vi "Telnet Parse AIC Command.vi"(11 "AIC sequence":string) -> (0 "error":bool, 1 "command":string, 2 "after sequence":string, 3 "AIC result":string, 4 "option negotiation":bool, 5 "sub option negotiation":bool, 6 "option info":T1)   [LabVIEW 2015, in "NI_InternetTK_Core_VIs.lvlib"]
uses:
  NI_InternetTK_Core_VIs.lvlib
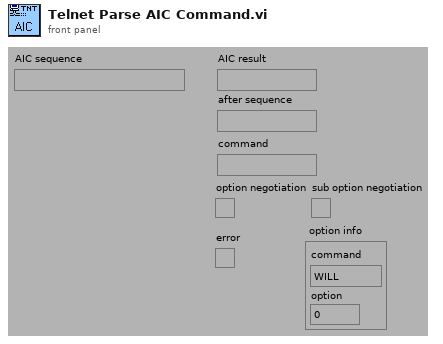
[diagram p1: front panel]
types:
  T1 = cluster{"command":enum16{"WILL", "WON'T", "DO", "DON'T"}, "option":u8}
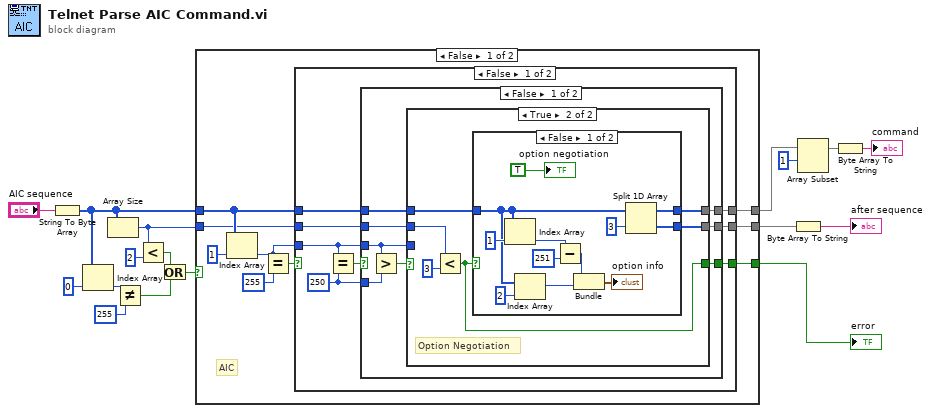
[diagram p0: block diagram]
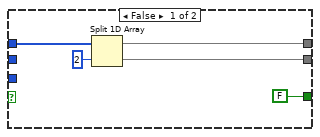
[diagram p2: hidden frame]
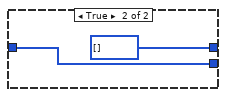
[diagram p3: hidden frame]
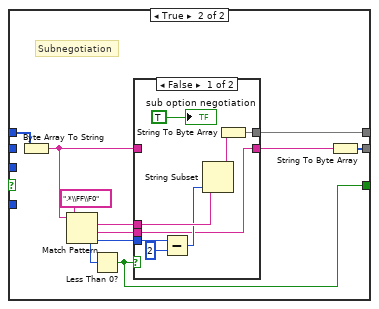
[diagram p4: hidden frame]
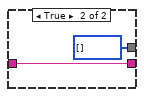
[diagram p5: hidden frame]
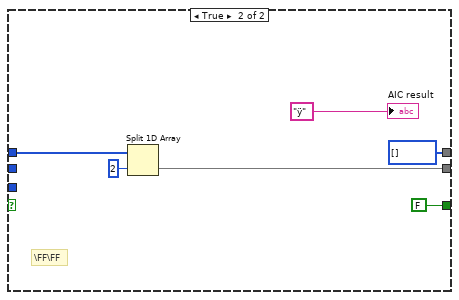
[diagram p6: hidden frame]
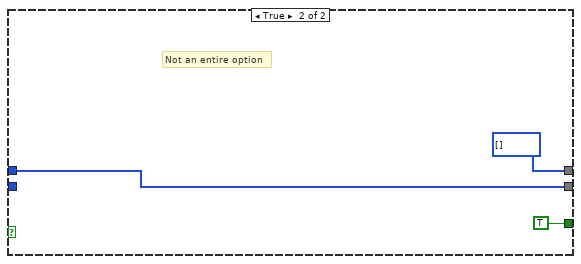
[diagram p7: hidden frame]
diagram:
  n1 = String To Byte Array(string="AIC sequence") -> (unsigned byte array=w15:u8[])
  n2 = Index Array(array=w15, index=0) -> (element=w13:u8)
  n3 = Array Size(array=w15) -> (size(s)=w5:i32)
  n4 = Not Equal?(x=w13, y=u8 255 ("x")) -> (x != y?=w12:bool)
  n5 = Less?(x=w5, y=2) -> (x < y?=w6:bool)
  n6 = Or(x=w6, y=w12) -> (x .or. y?=w7:bool)
  n7 = case shown="False" w7 {
    tunnel: w15 -> [w22 w95]
    tunnel: [w21 w95] -> w11
    tunnel: w5 -> [w20 _]
    tunnel: [w19 u8[] [] ("unsigned byte array")] -> w3
    tunnel: [w18 TRUE] -> w8
    frame False {
      # "AIC"
      n8 = Index Array(array=w22, index=1) -> (element=w24:u8)
      n9 = Equal?(x=w24, y=u8 255 ("x")) -> (x = y?=w23:bool)
      n10 = case shown="False" w23 {
        tunnel: w24 -> [w33 _]
        tunnel: w22 -> [w31 w93]
        tunnel: [w30 w91] -> w21
        tunnel: w20 -> [w29 _]
        tunnel: [w28 u8[] []] -> w19
        tunnel: [w27 FALSE] -> w18
        frame False {
          w34 = u8 250 ("x")
          n11 = Equal?(x=w33, y=w34) -> (x = y?=w32:bool)
          n12 = case shown="False" w32 {
            tunnel: w33 -> [w38 _]
            tunnel: w34 -> [w42 _]
            tunnel: w31 -> [w40 w77]
            tunnel: [w39 w75] -> w30
            tunnel: w29 -> [w37 _]
            tunnel: [w36 w69] -> w28
            tunnel: [w35 w68] -> w27
            frame False {
              n13 = Greater?(x=w38, y=w42) -> (0:w41:bool)
              n14 = case shown="True" w41 {
                tunnel: w40 -> [w47 w51]
                tunnel: [w45 w50] -> w39
                tunnel: w38 -> [_ _]
                tunnel: w37 -> [_ w52]
                tunnel: [w43 w49] -> w36
                tunnel: [FALSE w48] -> w35
                frame False {
                  n15 = Split 1D Array(array=w47, index=2) -> (first subarray=w43:u8[], second subarray=w45:u8[])
                }
                frame True {
                  # "Option Negotiation"
                  n16 = Less?(x=w52, y=3) -> (x < y?=w48:bool)
                  n17 = case shown="False" w48 {
                    tunnel: w51 -> [w55 w67]
                    tunnel: [w64 w67] -> w50
                    tunnel: [w63 u8[] []] -> w49
                    frame False {
                      n18 = Index Array(array=w55, index=1) -> (element=w60:u8)
                      n19 = Index Array(array=w55, index=2) -> (element=w54:u8)
                      n20 = Subtract(x=w60, y=u8 251) -> (x-y=w57:u8)
                      n21 = Bundle(w57, w54) -> (→"option info":cluster{u8, u8})  [unwired: 1 out]
                      n22 = Split 1D Array(array=w55, index=3) -> (first subarray=w63:u8[], second subarray=w64:u8[])
                      "option negotiation" <- TRUE ("option negotiation")
                    }
                    frame True {
                    }
                  }
                }
              }
            }
            frame True {
              # "Subnegotiation"
              n23 = Byte Array To String(unsigned byte array=w77) -> (string=w71:string)
              n24 = Match Pattern(string=w71, regular expression=".*\\FF\\F0") -> (match substring=w73:string, after substring=w70:string, offset past match=w74:i32)  [unwired: 2 out]
              n25 = Less Than 0?(x=w74) -> (x < 0?=w68:bool)
              n26 = case shown="False" w68 {
                tunnel: w73 -> [w85 _]
                tunnel: w74 -> [w84 _]
                tunnel: [w81 w87] -> w72
                tunnel: w71 -> [_ w87]
                tunnel: w70 -> [w81 _]
                tunnel: [w79 u8[] [] ("unsigned byte array")] -> w69
                frame False {
                  n27 = Subtract(x=w84, y=2) -> (x-y=w82:i32)
                  n28 = String Subset(string=w85, length (rest)=w82) -> (substring=w80:string)  [unwired: 1 out]
                  n29 = String To Byte Array(string=w80) -> (unsigned byte array=w79:u8[])
                  "sub option negotiation" <- TRUE ("sub option negotiation")
                }
                frame True {
                }
              }
              n30 = String To Byte Array(string=w72) -> (unsigned byte array=w75:u8[])
            }
          }
        }
        frame True {
          # "\\FF\\FF"
          n31 = Split 1D Array(array=w93, index=2) -> (second subarray=w91:u8[])  [unwired: 1 out]
          "AIC result" <- "ÿ" ("AIC result")
        }
      }
    }
    frame True {
      # "Not an entire option"
    }
  }
  "error" <- w8
  n32 = Byte Array To String(unsigned byte array=w11) -> (string=→"after sequence":string)
  n33 = Array Subset(array=w3, index=1) -> (w1:u8[])  [unwired: 1 in]
  n34 = Byte Array To String(unsigned byte array=w1) -> (string=→"command":string)
